vi "TL800_Driver.vi"(0 "Device In":refnum<visa-resource-name>="TL_Pro800", 5 "Commands":T1(ring)=enum."SET", 7 "Settings":T3={"Module"=2, "OnLineTEC"=23.2280006, "OnLineLD"=0.1722} {"OnLineLD" min=0.0 max=0.18 step=0.001 format="%.3p"; "OnLineTEC" min=16.0 max=28.0 step=0.1 format="%.3g"}, 11 "error in":errorcluster) -> (4 "Device Out":refnum<visa-resource-name>="Pro8000", 6 "Response":string, 8 "Readings":T2={"OnLineTEC"=23.2342777, "OnLineLD"=0.172234386, "OffLineTEC"=29.5498905, "OffLineLD"=0.17301172, "EtalonTEC"=27.0301247, "TSOA-TEC"=19.0111637, "Pro800"=TRUE, "OnLine TEC"=TRUE, "OnLine LD"=TRUE, "nothing"=TRUE, "nothing"=TRUE, "nothing"=TRUE, "nothing"=TRUE} {"OffLineLD" format="%.3p"; "OnLineLD" format="%.3p"; "TSOA-TEC" format="%.3g"; "EtalonTEC" format="%.3g"; "OffLineTEC" format="%.3g"; "OnLineTEC" format="%.3g"}, 15 "error out":errorcluster)   [LabVIEW 2012]
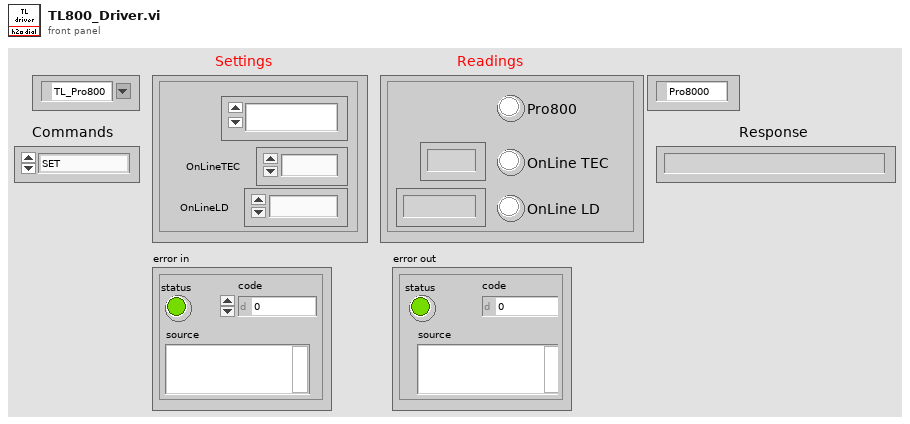
[diagram p1: front panel]
types:
  T1 = enum16{"Open_TL", "Close_TL", "Verify_ID", "TEC_Sensor", "SET", "READ", "ON", "OFF", "Read_Status"}
  T2 = cluster{"OnLineTEC":dbl, "OnLineLD":dbl, "OffLineTEC":dbl, "OffLineLD":dbl, "EtalonTEC":dbl, "TSOA-TEC":dbl, "Pro800":bool, "OnLine TEC":bool, "OnLine LD":bool, "nothing":bool, "nothing":bool, "nothing":bool, "nothing":bool}
  T3 = cluster{"Module":enum16{"On Line TEC", "On Line LD"}, "OnLineTEC":dbl, "OnLineLD":dbl}
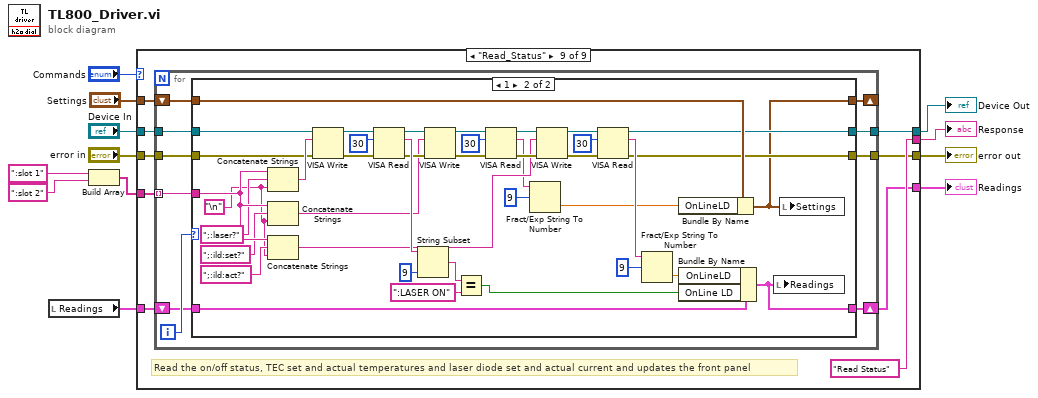
[diagram p0: block diagram]
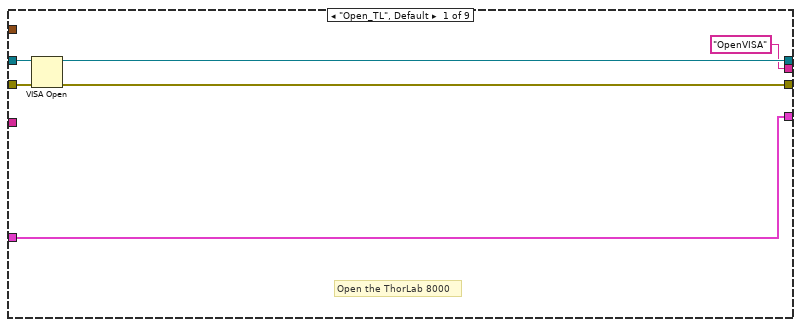
[diagram p2: hidden frame]
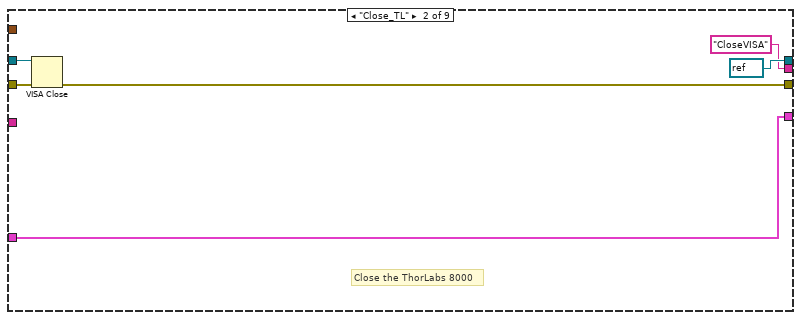
[diagram p3: hidden frame]
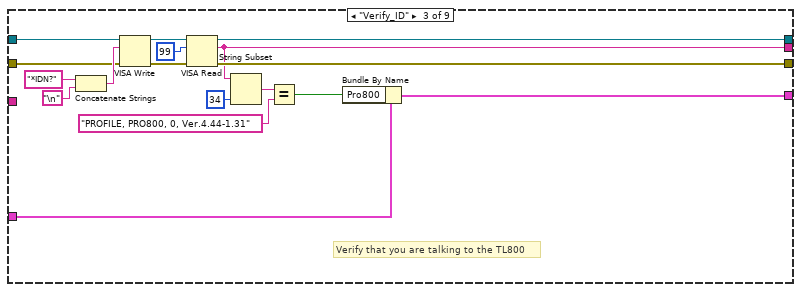
[diagram p4: hidden frame]
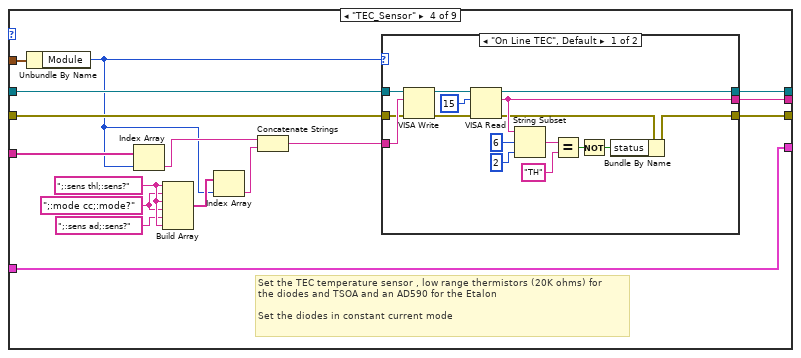
[diagram p5: hidden frame]
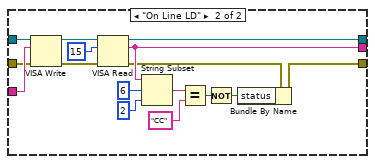
[diagram p6: hidden frame]
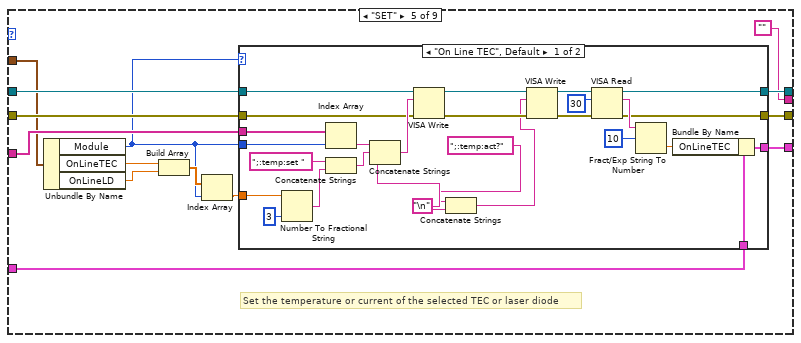
[diagram p7: hidden frame]
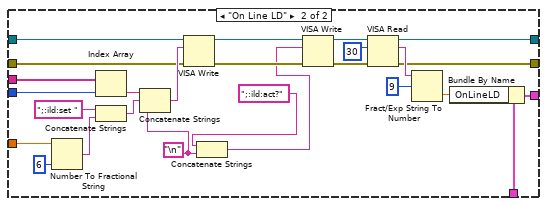
[diagram p8: hidden frame]
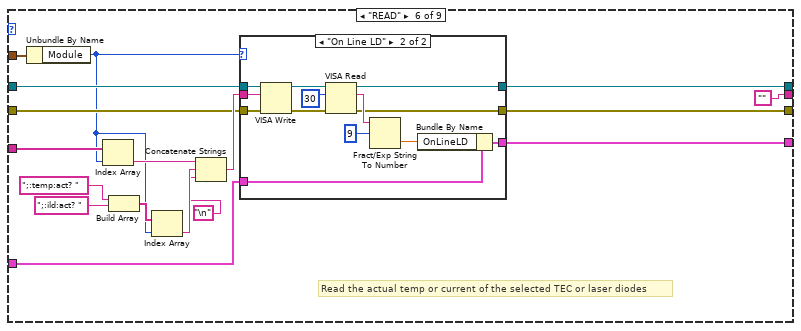
[diagram p9: hidden frame]
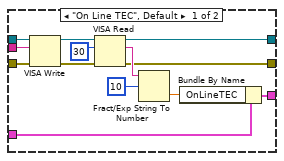
[diagram p10: hidden frame]
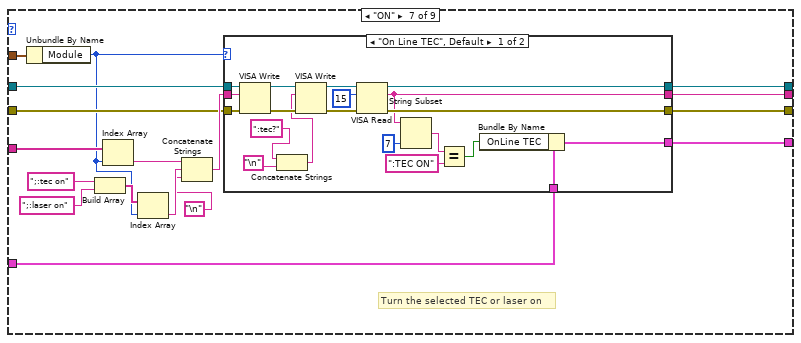
[diagram p11: hidden frame]
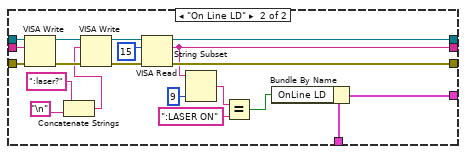
[diagram p12: hidden frame]
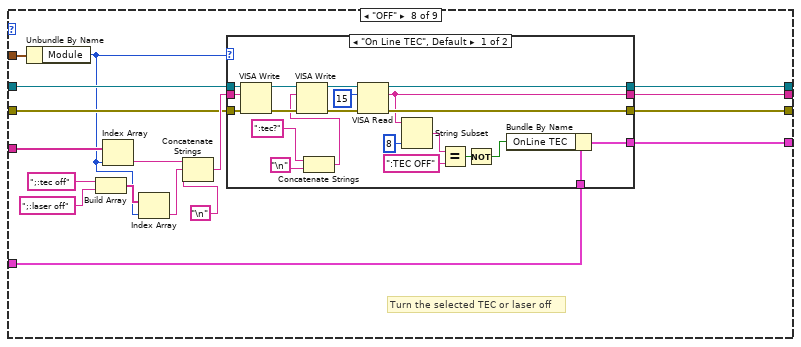
[diagram p13: hidden frame]
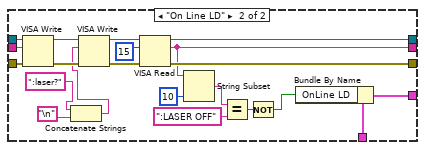
[diagram p14: hidden frame]
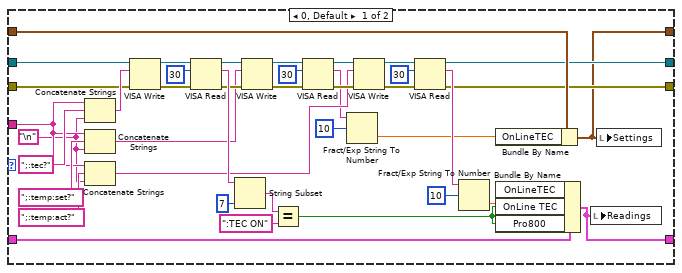
[diagram p15: hidden frame]
diagram:
  n1 = local read "Readings"() -> (w2:T2)
  n2 = Build Array(":slot 1", ":slot 2") -> (w9:string[])
  n3 = case shown="\"Read_Status\"" "Commands" {
    tunnel: "Device In" -> [w18 w24 w38 w56 w103 w171 w214 w271 w318]
    tunnel: "error in" -> [w17 w23 w35 w55 w102 w170 w213 w270 w321]
    tunnel: [w16 refnum<visa-resource-name> refnum ("VISA resource name") w33 w54 w99 w166 w210 w267 w319] -> w7
    tunnel: [w15 w22 w32 w51 w100 w165 w209 w266 w317] -> w11
    tunnel: ["OpenVISA" "CloseVISA" w31 w53 "" "" w208 w265 "Read Status"] -> w6
    tunnel: w9 -> [_ _ _ w50 w101 w168 w211 w268 w322]
    tunnel: "Settings" -> [_ _ _ w49 w97 w164 w207 w264 w320]
    tunnel: w2 -> [w13 w19 w27 w43 w91 w163 w206 w263 w316]
    tunnel: [w13 w19 w26 w43 w90 w162 w205 w262 w315] -> w1
    frame "Open_TL", Default {
      # "Open the ThorLab 8000"
      n4 = VISA Open(error in (no error)=w17, VISA resource name=w18) -> (VISA resource name=w16:refnum<visa-resource-name>, error out=w15:errorcluster)  [unwired: 3 in]
    }
    frame "Close_TL" {
      # "Close the ThorLabs 8000"
      n5 = VISA Close(VISA resource name=w24, error in (no error)=w23) -> (error out=w22:errorcluster)
    }
    frame "Verify_ID" {
      # "Verify that you are talking to the TL800"
      n6 = Concatenate Strings("*IDN?" ("string"), "\n") -> (w39:string)
      n7 = VISA Write(VISA resource name=w38, write buffer=w39, error in (no error)=w35) -> (VISA resource name out=w36:refnum<visa-resource-name>, error out=w34:errorcluster)  [unwired: 1 out]
      n8 = VISA Read(VISA resource name=w36, byte count=u32 99, error in (no error)=w34) -> (VISA resource name out=w33:refnum<visa-resource-name>, read buffer=w31:string, error out=w32:errorcluster)  [unwired: 1 out]
      n9 = String Subset(string=w31, length (rest)=34 ("length (rest)")) -> (substring=w29:string)  [unwired: 1 in]
      n10 = Equal?(x=w29, y="PROFILE, PRO800, 0, Ver.4.44-1.31" ("Response")) -> (x = y?=w25:bool)
      n11 = Bundle By Name(cluster=w27, "Pro800"=w25) -> (w26:T2)
    }
    frame "TEC_Sensor" {
      w42 = ";:mode cc;:mode?"
      w48 = ";:sens thl;:sens?" ("string")
      # "Set the TEC temperature sensor , low range thermistors (20K ohms) for\nthe diodes and TSOA and an AD590 for the Etalon\n\nSet the diodes in constant current mode"
      n12 = Unbundle By Name(w49) -> ("Module"=w44:enum16{"On Line TEC", "On Line LD"})
      n13 = Index Array(array=w50, index=w44) -> (element=w52:string)
      n14 = Build Array(w48, w42, w48, w42, ";:sens ad;:sens?" ("string"), w48) -> (w45:string[])
      n15 = Index Array(array=w45, index=w44) -> (element=w46:string)
      n16 = Concatenate Strings(w52, w46) -> (w57:string)
      n17 = case shown="\"On Line TEC\", Default" w44 {
        tunnel: w57 -> [w73 w89]
        tunnel: w56 -> [w72 w88]
        tunnel: w55 -> [w71 w87]
        tunnel: [w70 w86] -> w54
        tunnel: [w69 w85] -> w53
        tunnel: [w68 w84] -> w51
        frame "On Line TEC", Default {
          n18 = VISA Write(VISA resource name=w72, write buffer=w73, error in (no error)=w71) -> (VISA resource name out=w60:refnum<visa-resource-name>, error out=w59:errorcluster)  [unwired: 1 out]
          n19 = VISA Read(VISA resource name=w60, byte count=u32 15, error in (no error)=w59) -> (VISA resource name out=w70:refnum<visa-resource-name>, read buffer=w69:string, error out=w66:errorcluster)  [unwired: 1 out]
          n20 = String Subset(string=w69, offset (0)=6 ("length (rest)"), length (rest)=2 ("length (rest)")) -> (substring=w63:string)
          n21 = Equal?(x=w63, y="TH") -> (x = y?=w62:bool)
          n22 = Not(x=w62) -> (.not. x?=w61:bool)
          n23 = Bundle By Name(cluster=w66, "status"=w61) -> (w68:errorcluster)
        }
        frame "On Line LD" {
          n24 = VISA Write(VISA resource name=w88, write buffer=w89, error in (no error)=w87) -> (VISA resource name out=w76:refnum<visa-resource-name>, error out=w75:errorcluster)  [unwired: 1 out]
          n25 = VISA Read(VISA resource name=w76, byte count=u32 15, error in (no error)=w75) -> (VISA resource name out=w86:refnum<visa-resource-name>, read buffer=w85:string, error out=w82:errorcluster)  [unwired: 1 out]
          n26 = String Subset(string=w85, offset (0)=6 ("length (rest)"), length (rest)=2 ("length (rest)")) -> (substring=w79:string)
          n27 = Equal?(x=w79, y="CC") -> (x = y?=w78:bool)
          n28 = Not(x=w78) -> (.not. x?=w77:bool)
          n29 = Bundle By Name(cluster=w82, "status"=w77) -> (w84:errorcluster)
        }
      }
    }
    frame "SET" {
      # "Set the temperature or current of the selected TEC or laser diode"
      n30 = Unbundle By Name(w97) -> ("Module"=w94:enum16{"On Line TEC", "On Line LD"}, "OnLineTEC"=w93:dbl, "OnLineLD"=w92:dbl)
      n31 = Build Array(w93, w92) -> (w96:dbl[])
      n32 = Index Array(array=w96, index=w94) -> (element=w95:dbl)
      n33 = case shown="\"On Line TEC\", Default" w94 {
        tunnel: w103 -> [w128 w154]
        tunnel: w102 -> [w127 w153]
        tunnel: w101 -> [w125 w151]
        tunnel: [w110 w138] -> w100
        tunnel: [w109 w137] -> w99
        tunnel: w95 -> [w119 w145]
        tunnel: w94 -> [w120 w146]
        tunnel: w91 -> [w112 w136]
        tunnel: [w111 w135] -> w90
        frame "On Line TEC", Default {
          w106 = "\n"
          n34 = Number To Fractional String(number=w119, precision (6)=i16 3) -> (F-format string=w124:string)  [unwired: 2 in]
          n35 = Index Array(array=w125, index=w120) -> (element=w126:string)
          n36 = Concatenate Strings(";:temp:set " ("write buffer"), w124) -> (w121:string)
          n37 = Concatenate Strings(w126, w121, w106) -> (w129:string)
          n38 = VISA Write(VISA resource name=w128, write buffer=w129, error in (no error)=w127) -> (VISA resource name out=w108:refnum<visa-resource-name>, error out=w107:errorcluster)  [unwired: 1 out]
          n39 = Concatenate Strings(";:temp:act?" ("write buffer"), w106) -> (w104:string)
          n40 = VISA Write(VISA resource name=w108, write buffer=w104, error in (no error)=w107) -> (VISA resource name out=w114:refnum<visa-resource-name>, error out=w115:errorcluster)  [unwired: 1 out]
          n41 = VISA Read(VISA resource name=w114, byte count=u32 30, error in (no error)=w115) -> (VISA resource name out=w109:refnum<visa-resource-name>, read buffer=w116:string, error out=w110:errorcluster)  [unwired: 1 out]
          n42 = Fract/Exp String To Number(string=w116, offset=10) -> (number=w113:dbl)  [unwired: 2 in, 1 out]
          n43 = Bundle By Name(cluster=w112, "OnLineTEC"=w113) -> (w111:T2)
        }
        frame "On Line LD" {
          w132 = "\n"
          n44 = Number To Fractional String(number=w145, precision (6)=i16 6) -> (F-format string=w150:string)  [unwired: 2 in]
          n45 = Index Array(array=w151, index=w146) -> (element=w152:string)
          n46 = Concatenate Strings(";:ild:set " ("write buffer"), w150) -> (w147:string)
          n47 = Concatenate Strings(w152, w147, w132) -> (w155:string)
          n48 = VISA Write(VISA resource name=w154, write buffer=w155, error in (no error)=w153) -> (VISA resource name out=w134:refnum<visa-resource-name>, error out=w133:errorcluster)  [unwired: 1 out]
          n49 = Concatenate Strings(";:ild:act?" ("write buffer"), w132) -> (w130:string)
          n50 = VISA Write(VISA resource name=w134, write buffer=w130, error in (no error)=w133) -> (VISA resource name out=w140:refnum<visa-resource-name>, error out=w141:errorcluster)  [unwired: 1 out]
          n51 = VISA Read(VISA resource name=w140, byte count=u32 30, error in (no error)=w141) -> (VISA resource name out=w137:refnum<visa-resource-name>, read buffer=w142:string, error out=w138:errorcluster)  [unwired: 1 out]
          n52 = Fract/Exp String To Number(string=w142, offset=9) -> (number=w139:dbl)  [unwired: 2 in, 1 out]
          n53 = Bundle By Name(cluster=w136, "OnLineLD"=w139) -> (w135:T2)
        }
      }
    }
    frame "READ" {
      # "Read the actual temp or current of the selected TEC or laser diodes"
      n54 = Unbundle By Name(w164) -> ("Module"=w158:enum16{"On Line TEC", "On Line LD"})
      n55 = Index Array(array=w168, index=w158) -> (element=w169:string)
      n56 = Build Array(";:temp:act? " ("write buffer"), ";:ild:act? " ("write buffer")) -> (w159:string[])
      n57 = Index Array(array=w159, index=w158) -> (element=w157:string)
      n58 = Concatenate Strings(w169, w157, "\n") -> (w172:string)
      n59 = case shown="\"On Line LD\"" w158 {
        tunnel: w172 -> [w185 w198]
        tunnel: w171 -> [w184 w197]
        tunnel: w170 -> [w183 w196]
        tunnel: [w177 w190] -> w166
        tunnel: [w176 w189] -> w165
        tunnel: w163 -> [w174 w187]
        tunnel: [w173 w186] -> w162
        frame "On Line TEC", Default {
          n60 = VISA Write(VISA resource name=w184, write buffer=w185, error in (no error)=w183) -> (VISA resource name out=w178:refnum<visa-resource-name>, error out=w179:errorcluster)  [unwired: 1 out]
          n61 = VISA Read(VISA resource name=w178, byte count=u32 30, error in (no error)=w179) -> (VISA resource name out=w177:refnum<visa-resource-name>, read buffer=w180:string, error out=w176:errorcluster)  [unwired: 1 out]
          n62 = Fract/Exp String To Number(string=w180, offset=10) -> (number=w175:dbl)  [unwired: 2 in, 1 out]
          n63 = Bundle By Name(cluster=w174, "OnLineTEC"=w175) -> (w173:T2)
        }
        frame "On Line LD" {
          n64 = VISA Write(VISA resource name=w197, write buffer=w198, error in (no error)=w196) -> (VISA resource name out=w191:refnum<visa-resource-name>, error out=w192:errorcluster)  [unwired: 1 out]
          n65 = VISA Read(VISA resource name=w191, byte count=u32 30, error in (no error)=w192) -> (VISA resource name out=w190:refnum<visa-resource-name>, read buffer=w193:string, error out=w189:errorcluster)  [unwired: 1 out]
          n66 = Fract/Exp String To Number(string=w193, offset=9) -> (number=w188:dbl)  [unwired: 2 in, 1 out]
          n67 = Bundle By Name(cluster=w187, "OnLineLD"=w188) -> (w186:T2)
        }
      }
    }
    frame "ON" {
      # "Turn the selected TEC or laser on"
      n68 = Unbundle By Name(w207) -> ("Module"=w201:enum16{"On Line TEC", "On Line LD"})
      n69 = Build Array(";:tec on" ("write buffer"), ";:laser on" ("write buffer")) -> (w203:string[])
      n70 = Index Array(array=w211, index=w201) -> (element=w212:string)
      n71 = Index Array(array=w203, index=w201) -> (element=w200:string)
      n72 = Concatenate Strings(w212, w200, "\n") -> (w215:string)
      n73 = case shown="\"On Line TEC\", Default" w201 {
        tunnel: w215 -> [w235 w255]
        tunnel: w214 -> [w234 w254]
        tunnel: w213 -> [w233 w253]
        tunnel: [w231 w251] -> w210
        tunnel: [w230 w250] -> w209
        tunnel: [w222 w242] -> w208
        tunnel: w206 -> [w221 w241]
        tunnel: [w220 w240] -> w205
        frame "On Line TEC", Default {
          n74 = VISA Write(VISA resource name=w234, write buffer=w235, error in (no error)=w233) -> (VISA resource name out=w227:refnum<visa-resource-name>, error out=w229:errorcluster)  [unwired: 1 out]
          n75 = Concatenate Strings(":tec?" ("write buffer"), "\n") -> (w216:string)
          n76 = VISA Write(VISA resource name=w227, write buffer=w216, error in (no error)=w229) -> (VISA resource name out=w226:refnum<visa-resource-name>, error out=w228:errorcluster)  [unwired: 1 out]
          n77 = VISA Read(VISA resource name=w226, byte count=u32 15, error in (no error)=w228) -> (VISA resource name out=w231:refnum<visa-resource-name>, read buffer=w222:string, error out=w230:errorcluster)  [unwired: 1 out]
          n78 = String Subset(string=w222, length (rest)=7 ("offset (0)")) -> (substring=w224:string)  [unwired: 1 in]
          n79 = Equal?(x=w224, y=":TEC ON") -> (x = y?=w219:bool)
          n80 = Bundle By Name(cluster=w221, "OnLine TEC"=w219) -> (w220:T2)
        }
        frame "On Line LD" {
          n81 = VISA Write(VISA resource name=w254, write buffer=w255, error in (no error)=w253) -> (VISA resource name out=w247:refnum<visa-resource-name>, error out=w249:errorcluster)  [unwired: 1 out]
          n82 = Concatenate Strings(":laser?" ("write buffer"), "\n") -> (w236:string)
          n83 = VISA Write(VISA resource name=w247, write buffer=w236, error in (no error)=w249) -> (VISA resource name out=w246:refnum<visa-resource-name>, error out=w248:errorcluster)  [unwired: 1 out]
          n84 = VISA Read(VISA resource name=w246, byte count=u32 15, error in (no error)=w248) -> (VISA resource name out=w251:refnum<visa-resource-name>, read buffer=w242:string, error out=w250:errorcluster)  [unwired: 1 out]
          n85 = String Subset(string=w242, length (rest)=9 ("offset (0)")) -> (substring=w244:string)  [unwired: 1 in]
          n86 = Equal?(x=w244, y=":LASER ON") -> (x = y?=w239:bool)
          n87 = Bundle By Name(cluster=w241, "OnLine LD"=w239) -> (w240:T2)
        }
      }
    }
    frame "OFF" {
      # "Turn the selected TEC or laser off"
      n88 = Unbundle By Name(w264) -> ("Module"=w257:enum16{"On Line TEC", "On Line LD"})
      n89 = Build Array(";:tec off" ("write buffer"), ";:laser off" ("write buffer")) -> (w259:string[])
      n90 = Index Array(array=w268, index=w257) -> (element=w269:string)
      n91 = Index Array(array=w259, index=w257) -> (element=w258:string)
      n92 = Concatenate Strings(w269, w258, "\n") -> (w272:string)
      n93 = case shown="\"On Line TEC\", Default" w257 {
        tunnel: w272 -> [w293 w314]
        tunnel: w271 -> [w292 w313]
        tunnel: w270 -> [w291 w312]
        tunnel: [w289 w310] -> w267
        tunnel: [w288 w309] -> w266
        tunnel: [w280 w301] -> w265
        tunnel: w263 -> [w279 w300]
        tunnel: [w278 w299] -> w262
        frame "On Line TEC", Default {
          n94 = VISA Write(VISA resource name=w292, write buffer=w293, error in (no error)=w291) -> (VISA resource name out=w285:refnum<visa-resource-name>, error out=w287:errorcluster)  [unwired: 1 out]
          n95 = Concatenate Strings(":tec?" ("write buffer"), "\n") -> (w273:string)
          n96 = VISA Write(VISA resource name=w285, write buffer=w273, error in (no error)=w287) -> (VISA resource name out=w284:refnum<visa-resource-name>, error out=w286:errorcluster)  [unwired: 1 out]
          n97 = VISA Read(VISA resource name=w284, byte count=u32 15, error in (no error)=w286) -> (VISA resource name out=w289:refnum<visa-resource-name>, read buffer=w280:string, error out=w288:errorcluster)  [unwired: 1 out]
          n98 = String Subset(string=w280, length (rest)=8 ("offset (0)")) -> (substring=w282:string)  [unwired: 1 in]
          n99 = Equal?(x=w282, y=":TEC OFF") -> (x = y?=w277:bool)
          n100 = Not(x=w277) -> (.not. x?=w276:bool)
          n101 = Bundle By Name(cluster=w279, "OnLine TEC"=w276) -> (w278:T2)
        }
        frame "On Line LD" {
          n102 = VISA Write(VISA resource name=w313, write buffer=w314, error in (no error)=w312) -> (VISA resource name out=w306:refnum<visa-resource-name>, error out=w308:errorcluster)  [unwired: 1 out]
          n103 = Concatenate Strings(":laser?" ("write buffer"), "\n") -> (w294:string)
          n104 = VISA Write(VISA resource name=w306, write buffer=w294, error in (no error)=w308) -> (VISA resource name out=w305:refnum<visa-resource-name>, error out=w307:errorcluster)  [unwired: 1 out]
          n105 = VISA Read(VISA resource name=w305, byte count=u32 15, error in (no error)=w307) -> (VISA resource name out=w310:refnum<visa-resource-name>, read buffer=w301:string, error out=w309:errorcluster)  [unwired: 1 out]
          n106 = String Subset(string=w301, length (rest)=10 ("offset (0)")) -> (substring=w303:string)  [unwired: 1 in]
          n107 = Equal?(x=w303, y=":LASER OFF") -> (x = y?=w298:bool)
          n108 = Not(x=w298) -> (.not. x?=w297:bool)
          n109 = Bundle By Name(cluster=w300, "OnLine LD"=w297) -> (w299:T2)
        }
      }
    }
    frame "Read_Status" {
      # "Read the on/off status, TEC set and actual temperatures and laser diode set and actual current and updates the front panel"
      n110 = for {
        tunnel: w322 -> [w330] mode=indexing
        tunnel: w321 -> [w331]
        tunnel: [w326] -> w317
        tunnel: w318 -> [w327]
        tunnel: [w328] -> w319
        shift-right: [w325] -> w315
        shift-left: w316 -> [w332]
        shift-right: [w324] -> _
        shift-left: w320 -> [w329]
        i -> [w333]
        n111 = case shown="1" w333 {
          tunnel: w332 -> [w347 w390]
          tunnel: w327 -> [w350 w393]
          tunnel: w331 -> [w349 w392]
          tunnel: w330 -> [w348 w391]
          tunnel: w329 -> [w344 w386]
          tunnel: [w339 w381] -> w328
          tunnel: [w338 w380] -> w326
          tunnel: [w336 w375] -> w325
          tunnel: [w337 w376] -> w324
          frame 0, Default {
            w334 = "\n"
            n112 = Concatenate Strings(w348, ";:tec?" ("write buffer"), w334) -> (w370:string)
            n113 = Concatenate Strings(w348, ";:temp:set?" ("write buffer"), w334) -> (w357:string)
            n114 = Concatenate Strings(w348, ";:temp:act?" ("write buffer"), w334) -> (w352:string)
            n115 = VISA Write(VISA resource name=w350, write buffer=w370, error in (no error)=w349) -> (VISA resource name out=w371:refnum<visa-resource-name>, error out=w372:errorcluster)  [unwired: 1 out]
            n116 = VISA Read(VISA resource name=w371, byte count=u32 30, error in (no error)=w372) -> (VISA resource name out=w361:refnum<visa-resource-name>, read buffer=w365:string, error out=w360:errorcluster)  [unwired: 1 out]
            n117 = String Subset(string=w365, length (rest)=7 ("offset (0)")) -> (substring=w367:string)  [unwired: 1 in]
            n118 = VISA Write(VISA resource name=w361, write buffer=w357, error in (no error)=w360) -> (VISA resource name out=w362:refnum<visa-resource-name>, error out=w363:errorcluster)  [unwired: 1 out]
            n119 = Equal?(x=w367, y=":TEC ON") -> (x = y?=w335:bool)
            n120 = VISA Read(VISA resource name=w362, byte count=u32 30, error in (no error)=w363) -> (VISA resource name out=w353:refnum<visa-resource-name>, read buffer=w345:string, error out=w354:errorcluster)  [unwired: 1 out]
            n121 = Fract/Exp String To Number(string=w345, offset=10) -> (number=w340:dbl)  [unwired: 2 in, 1 out]
            n122 = VISA Write(VISA resource name=w353, write buffer=w352, error in (no error)=w354) -> (VISA resource name out=w355:refnum<visa-resource-name>, error out=w351:errorcluster)  [unwired: 1 out]
            n123 = VISA Read(VISA resource name=w355, byte count=u32 30, error in (no error)=w351) -> (VISA resource name out=w339:refnum<visa-resource-name>, read buffer=w342:string, error out=w338:errorcluster)  [unwired: 1 out]
            n124 = Fract/Exp String To Number(string=w342, offset=10) -> (number=w341:dbl)  [unwired: 2 in, 1 out]
            n125 = Bundle By Name(cluster=w344, "OnLineTEC"=w340) -> (w337:T3)
            n126 = Bundle By Name(cluster=w347, "OnLineTEC"=w341, "OnLine TEC"=w335, "Pro800"=w335) -> (w336:T2)
            n127 = local write "Readings"(w336) -> ()
            n128 = local write "Settings"(w337) -> ()
          }
          frame 1 {
            w374 = "\n"
            n129 = Concatenate Strings(w391, ";:laser?" ("write buffer"), w374) -> (w410:string)
            n130 = Concatenate Strings(w391, ";:ild:set?" ("write buffer"), w374) -> (w400:string)
            n131 = Concatenate Strings(w391, ";:ild:act?" ("write buffer"), w374) -> (w395:string)
            n132 = VISA Write(VISA resource name=w393, write buffer=w410, error in (no error)=w392) -> (VISA resource name out=w411:refnum<visa-resource-name>, error out=w412:errorcluster)  [unwired: 1 out]
            n133 = VISA Read(VISA resource name=w411, byte count=u32 30, error in (no error)=w412) -> (VISA resource name out=w402:refnum<visa-resource-name>, read buffer=w406:string, error out=w401:errorcluster)  [unwired: 1 out]
            n134 = String Subset(string=w406, length (rest)=9 ("offset (0)")) -> (substring=w408:string)  [unwired: 1 in]
            n135 = VISA Write(VISA resource name=w402, write buffer=w400, error in (no error)=w401) -> (VISA resource name out=w403:refnum<visa-resource-name>, error out=w404:errorcluster)  [unwired: 1 out]
            n136 = Equal?(x=w408, y=":LASER ON") -> (x = y?=w389:bool)
            n137 = VISA Read(VISA resource name=w403, byte count=u32 30, error in (no error)=w404) -> (VISA resource name out=w396:refnum<visa-resource-name>, read buffer=w387:string, error out=w397:errorcluster)  [unwired: 1 out]
            n138 = Fract/Exp String To Number(string=w387, offset=9) -> (number=w382:dbl)  [unwired: 2 in, 1 out]
            n139 = VISA Write(VISA resource name=w396, write buffer=w395, error in (no error)=w397) -> (VISA resource name out=w398:refnum<visa-resource-name>, error out=w394:errorcluster)  [unwired: 1 out]
            n140 = VISA Read(VISA resource name=w398, byte count=u32 30, error in (no error)=w394) -> (VISA resource name out=w381:refnum<visa-resource-name>, read buffer=w384:string, error out=w380:errorcluster)  [unwired: 1 out]
            n141 = Fract/Exp String To Number(string=w384, offset=9) -> (number=w383:dbl)  [unwired: 2 in, 1 out]
            n142 = Bundle By Name(cluster=w386, "OnLineLD"=w382) -> (w376:T3)
            n143 = Bundle By Name(cluster=w390, "OnLineLD"=w383, "OnLine LD"=w389) -> (w375:T2)
            n144 = local write "Readings"(w375) -> ()
            n145 = local write "Settings"(w376) -> ()
          }
        }
      }
    }
  }
  "error out" <- w11
  "Device Out" <- w7
  "Response" <- w6
  "Readings" <- w1
